vi "CRYPlot Polar Data.vi"(0 "picture":picture, 5 "polar data":cluster{"magnitude":dbl, "phase":dbl}[](array[cluster]) {"phase" format="%0.2f"; "magnitude" format="%0.2f"}, 7 "grid measurements":T2 {"end angle" format="%0.2f"; "start angle" format="%0.2f"; "scale factors"."b" format="%0.2f"; "scale factors"."a" format="%0.2f"}, 9 "polar attributes":T3 {"minimum" format="%0.2f"; "maximum" format="%0.2f"}, 11 "pen":T1={"Width"=1, "Style"=enum."Solid"}) -> (4 "new picture":picture)   [LabVIEW 2013]
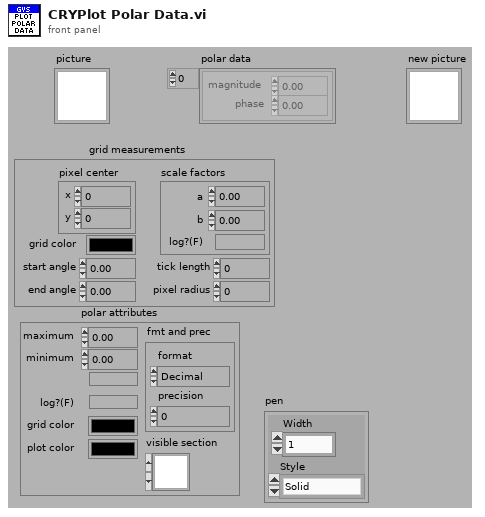
[diagram p1: front panel]
types:
  T1 = cluster{"Width":u16, "Style":enum32{"Solid", "Dash", "Dot", "DashDot", "DashDotDot"}}
  T2 = cluster{"pixel center":cluster{"x":i16, "y":i16}, "scale factors":cluster{"a":dbl, "b":dbl, "log?(F)":bool}, "grid color":u32, "start angle":dbl, "end angle":dbl, "tick length":i16, "pixel radius":i32}
  T3 = cluster{"maximum":dbl, "minimum":dbl, "clip to min":bool, "log?(F)":bool, "grid color":u32, "plot color":u32, "fmt and prec":cluster{"format":enum8{"Decimal", "Scientific", "Engineering", "Binary", "Octal", "Hex"}, "precision":u8}, "visible section":u16}
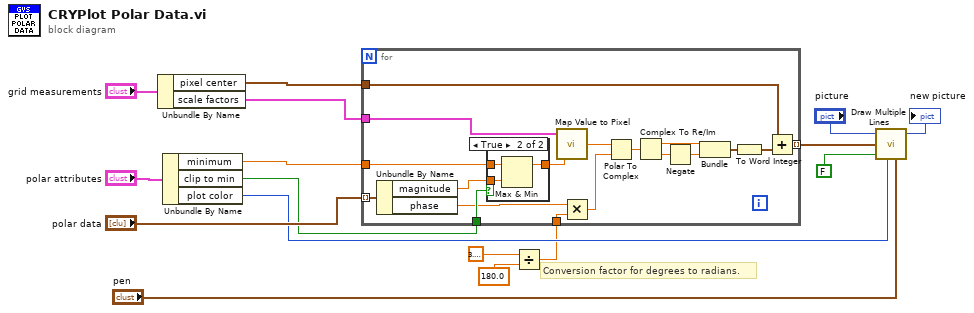
[diagram p0: block diagram]
diagram:
  # "Conversion factor for degrees to radians."
  n1 = Unbundle By Name("grid measurements") -> ("pixel center"=w8:cluster{"x":i16, "y":i16}, "scale factors"=w9:cluster{"a":dbl, "b":dbl, "log?(F)":bool})
  n2 = Unbundle By Name("polar attributes") -> ("minimum"=w7:dbl, "clip to min"=w5:bool, "plot color"=w6:u32)
  n3 = Divide(x=3.141592653589793, y=180.0) -> (x/y=w3:dbl)
  n4 = for {
    tunnel: "polar data" -> [w34] mode=indexing
    tunnel: w8 -> [w33]
    tunnel: [w32] -> w12 mode=indexing
    tunnel: w9 -> [w25]
    tunnel: w7 -> [w21]
    tunnel: w5 -> [w20]
    tunnel: w3 -> [w17]
    n5 = Unbundle By Name(w34) -> ("magnitude"=w22:dbl, "phase"=w18:dbl)
    n6 = case shown="True" w20 {
      tunnel: w22 -> [w35 w38]
      tunnel: [w35 w37] -> w23
      tunnel: w21 -> [_ w36]
      frame False {
      }
      frame True {
        n7 = Max & Min(x=w36, y=w38) -> (max(x,y)=w37:dbl)  [unwired: 1 out]
      }
    }
    n8 = call <vilib>:"Map Value to Pixel.vi"("x"=w23, "scale factors"=w25) -> ("pixel"=w24:dbl)  [unwired: 1 in]
    n9 = Multiply(x=w18, y=w17) -> (x*y=w19:dbl)
    n10 = Polar To Complex(1:w19, 2:w24) -> (0:w31:cdb)
    n11 = Complex To Re/Im(x + iy=w31) -> (x=w29:dbl, y=w28:dbl)
    n12 = Negate(x=w28) -> (-x=w26:dbl)
    n13 = Bundle(w29, w26) -> (w30:cluster{dbl, dbl})  [unwired: 1 in]
    n14 = To Word Integer(number=w30) -> (16bit integer=w27:cluster{i16, i16})
    n15 = Add(x=w33, y=w27) -> (x+y=w32:cluster{i16, i16})
  }
  n16 = call <vilib>:"Draw Multiple Lines.vi"("picture"="picture", "line endpoints"=w12, "fill?(F)"=FALSE, "color(black)"=w6, "pen"="pen") -> ("new picture"=→"new picture":picture)  [unwired: 4 in]
